vi "Configure Multicolumn Listbox for Displayed Channels.vi"(4 "table values":T1, 5 "widest value strings":string[](array[string]), 9 "MulticolumnListbox in":refnum<vi>) -> ()   [LabVIEW 2020, in "TdmsFileViewer.lvlib"]
uses:
  TdmsFileViewer.lvlib
  Table Components.ctl
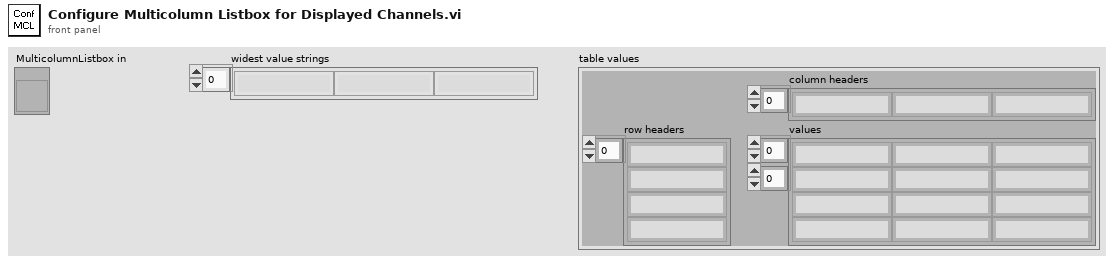
[diagram p1: front panel]
types:
  T1 = typedef "TdmsFileViewer.lvlib/Table Components.ctl" = cluster{"column headers":string[], "row headers":string[], "values":string[][]}
  T2 = typedef "LVRowAndColumnUnsignedTypeDef.ctl" = cluster{"Row":u32, "Column":u32}
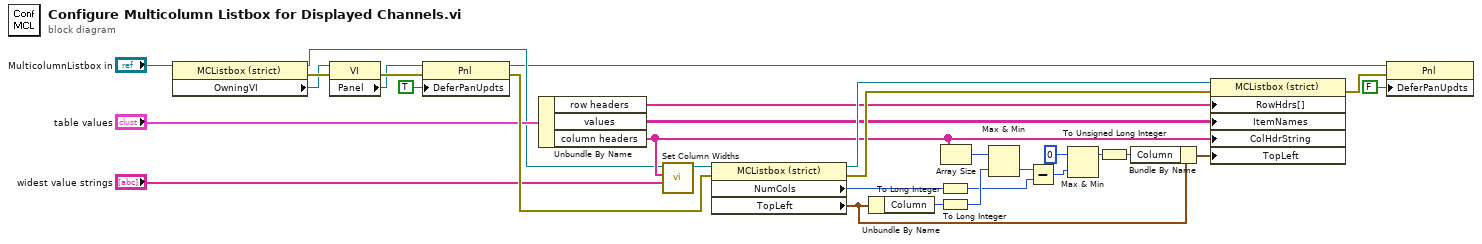
[diagram p0: block diagram]
diagram:
  n1 = property class="MCListbox (strict)"(reference="MulticolumnListbox in") -> (reference out=w3:refnum<vi>, error out=w31:errorcluster, "OwningVI"=w7:refnum<vi>)  [unwired: 1 in]
  n2 = property class="VI"(reference=w7, error in=w31) -> (error out=w30:errorcluster, "Panel"=w6:refnum<vi>)  [unwired: 1 out]
  n3 = property class="Pnl"(reference=w6, error in=w30, "DeferPanUpdts"=TRUE ("Defer Panel Updates")) -> (reference out=w1:refnum<vi>, error out=w28:errorcluster)
  n4 = Unbundle By Name("table values") -> ("row headers"=w12:string[], "values"=w11:string[][], "column headers"=w8:string[])
  n5 = call "Set Column Widths.vi"("widest value strings"="widest value strings", "column headers"=w8, "MulticolumnListbox in"=w3) -> ("MulticolumnListbox out"=w10:refnum<vi>)  [unwired: 8 in]
  n6 = property on="Property Node" class="MCListbox (strict)"(reference=w10, error in=w28) -> (reference out=w14:refnum<vi>, error out=w27:errorcluster, "NumCols"=w23:u32, "TopLeft"=w21:T2)
  n7 = Unbundle By Name(w21) -> ("Column"=w19:u32)
  n8 = To Long Integer(number=w23) -> (32bit integer=w24:i32)
  n9 = To Long Integer(number=w19) -> (32bit integer=w25:i32)
  n10 = Array Size(array=w8) -> (size(s)=w18:i32)
  n11 = Max & Min(x=w18, y=w25) -> (min(x,y)=w17:i32)  [unwired: 1 out]
  n12 = Subtract(x=w17, y=w24) -> (x-y=w15:i32)
  n13 = Max & Min(x=0 ("y"), y=w15) -> (max(x,y)=w20:i32)  [unwired: 1 out]
  n14 = To Unsigned Long Integer(number=w20) -> (unsigned 32bit integer=w26:u32)
  n15 = Bundle By Name(cluster=w21, "Column"=w26) -> (w22:T2)
  n16 = property on="Property Node" class="MCListbox (strict)"(reference=w14, error in=w27, "RowHdrs[]"=w12, "ItemNames"=w11, "ColHdrString"=w8, "TopLeft"=w22) -> (error out=w29:errorcluster)  [unwired: 1 out]
  n17 = property class="Pnl"(reference=w1, error in=w29, "DeferPanUpdts"=FALSE ("Defer Panel Updates")) -> ()  [unwired: 2 out]
